vi "Remove Channel.vi"(6 "Index from Loop Node (0)":i32, 8 "error in (no error)":errorcluster, 10 "Name List":string[](array[string]), 11 "ChannelVS in":refnum<class "ChannelVS.lvclass">) -> (0 "error out":errorcluster, 2 "Cancelled":bool)   [LabVIEW 2017, in "Shared Variables CD 2.0 Configuration.lvlib" / "ChannelVS.lvclass"]
doc: "When Index is not connected and VI is used in a loop, delete confirmation message shows for each channel. Connect Index Control from loop to only show message once."
uses:
  ChannelVS.lvclass
  ChannelVS.lvclass/ChannelVS.ctl
  Shared/SV Global.vi
  <vilib>/NI Veristand/Custom Device API/Get Item Property (String).vi
  <vilib>/NI VeriStand/Custom Device API/Custom Device API.lvlib
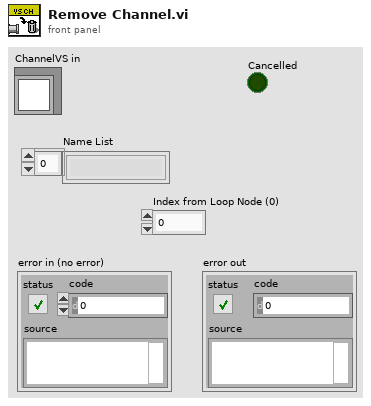
[diagram p1: front panel]
types:
  T1 = typedef "Custom Device API.lvlib/Custom Device Item Ref.ctl" = u64
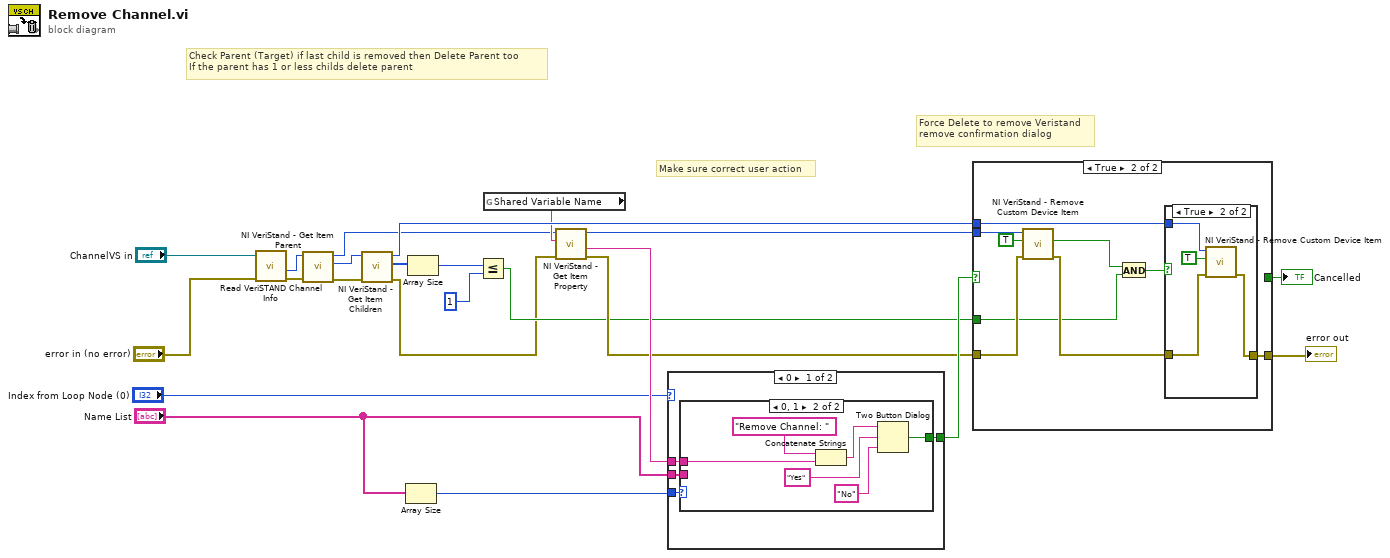
[diagram p0: block diagram]
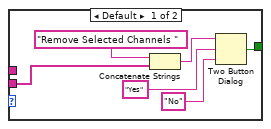
[diagram p2: hidden frame]
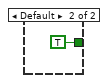
[diagram p3: hidden frame]
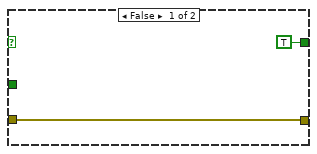
[diagram p4: hidden frame]
diagram:
  # "Force Delete to remove Veristand\nremove confirmation dialog"
  # "Make sure correct user action"
  # "Check Parent (Target) if last child is removed then Delete Parent too\nIf the parent has 1 or less childs delete parent"
  n1 = call "Read VeriSTAND Channel Info.vi"("error in (no error)"="error in (no error)", "ChannelVS in"="ChannelVS in") -> ("error out"=w4:errorcluster, "VeriSTAND Reference"=w3:T1)  [unwired: 6 in, 2 out]
  n2 = call <vilib>:"NI VeriStand - Get Item Parent.vi"("error in (no error)"=w4, "Item Ref in"=w3) -> ("error out"=w12:errorcluster, "Parent Ref"=w6:T1, "Item Ref out"=w5:T1)  [unwired: 6 in, 1 out]
  n3 = call <vilib>:"NI VeriStand - Get Item Children.vi"("error in (no error)"=w12, "Item Ref in"=w6) -> ("error out"=w15:errorcluster, "Child Refs"=w14:T1[], "Item Ref out"=w20:T1)  [unwired: 6 in, 1 out]
  n4 = Array Size(array="Name List") -> (size(s)=w8:i32)
  n5 = Array Size(array=w14) -> (size(s)=w16:i32)
  n6 = Less Or Equal?(x=w16, y=1) -> (x <= y?=w19:bool)
  n7 = global read "SV Global.vi" "Shared Variable Name"() -> (w13:string)
  n8 = call-poly <vilib>:"NI VeriStand - Get Item Property.vi"("error in (no error)"=w15, "Property Name"=w13, "Item Ref in"=w5) -> ("error out"=w21:errorcluster, "Value"=w22:string, "Item Ref out"=w18:T1)  [unwired: 5 in, 1 out]
  n9 = case shown="0" "Index from Loop Node (0)" {
    tunnel: [w27 TRUE ("T button?")] -> w23
    tunnel: w22 -> [w26 _]
    tunnel: "Name List" -> [w25 _]
    tunnel: w8 -> [w24 _]
    frame 0 {
      n10 = case shown="0, 1" w24 {
        tunnel: [w29 w39] -> w27
        tunnel: w26 -> [_ w38]
        tunnel: w25 -> [w28 _]
        frame Default {
          n11 = Concatenate Strings("Remove Selected Channels " ("message"), w28) -> (w33:string)
          n12 = Two Button Dialog(message=w33, 1:"No" ("F button name (\"Cancel\")"), 2:"Yes" ("T button name (\"OK\")")) -> (T button?=w29:bool)
        }
        frame 0, 1 {
          n13 = Concatenate Strings("Remove Channel: " ("message"), w38) -> (w36:string)
          n14 = Two Button Dialog(message=w36, 1:"No" ("F button name (\"Cancel\")"), 2:"Yes" ("T button name (\"OK\")")) -> (T button?=w39:bool)
        }
      }
    }
    frame Default {
    }
  }
  n15 = case shown="True" w23 {
    tunnel: [w42 w51] -> w11
    tunnel: w18 -> [_ w50]
    tunnel: w21 -> [w42 w49]
    tunnel: w19 -> [_ w46]
    tunnel: w20 -> [_ w44]
    tunnel: [TRUE _] -> w10
    frame False {
    }
    frame True {
      n16 = call <vilib>:"NI VeriStand - Remove Custom Device Item.vi"("error in (no error)"=w49, "Force Delete (F)"=TRUE, "Item Ref in"=w50) -> ("error out"=w48:errorcluster, "Deleted?"=w47:bool)  [unwired: 7 in]
      n17 = And(x=w47, y=w46) -> (x .and. y?=w45:bool)
      n18 = case shown="True" w45 {
        tunnel: [w52 w56] -> w51
        tunnel: w48 -> [w52 w55]
        tunnel: w44 -> [_ w53]
        frame False {
        }
        frame True {
          n19 = call <vilib>:"NI VeriStand - Remove Custom Device Item.vi"("error in (no error)"=w55, "Force Delete (F)"=TRUE, "Item Ref in"=w53) -> ("error out"=w56:errorcluster)  [unwired: 7 in, 1 out]
        }
      }
    }
  }
  "error out" <- w11
  "Cancelled" <- w10
